vi "Get sub-Array by names.vi"(8 "error in (no error)":errorcluster, 10 "Name Array":string[](array[string]), 11 "JSON Value In":refnum<class "JSON Value.lvclass">) -> (0 "error out":errorcluster, 1 "found":bool, 2 "Array":refnum<class "JSON Value.lvclass">[](array[class]), 3 "JSON Value Out":refnum<class "JSON Value.lvclass">)   [LabVIEW 2020, in "Library Commun.lvlib" / "JSON Value.lvclass"]
doc: "Gets a JSON object from a JSON collection by it's path (an array of strings).\n\nCopyright 2012 James David Powell, Shaun Rumbell and Ton Plomp\nMore information on http://lavag.org/topic/16217-cr-json-labview"
uses:
  JSON Value.lvclass
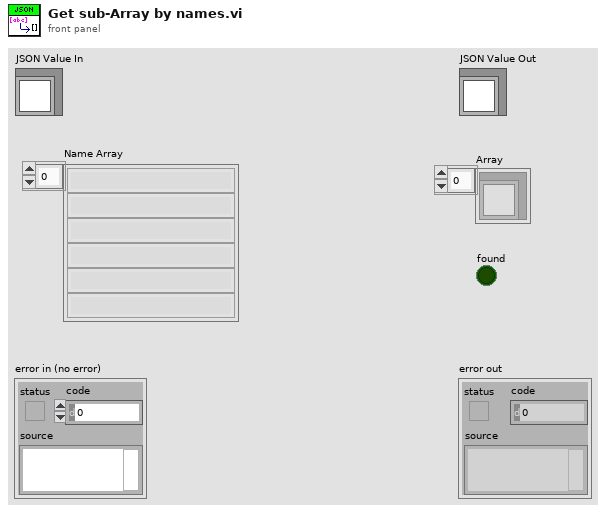
[diagram p1: front panel]
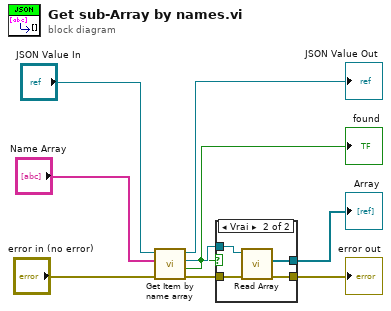
[diagram p0: block diagram]
diagram:
  n1 = call "Get Item by name array.vi"("error in (no error)"="error in (no error)", "Name Array"="Name Array", "JSON Value In"="JSON Value In") -> ("error out"=w2:errorcluster, "found"=w4:bool, "Value"=w5:refnum<class "JSON Value.lvclass">, "JSON Value Out"=→"JSON Value Out":refnum<class "JSON Value.lvclass">)  [unwired: 5 in]
  "found" <- w4
  n2 = case shown="Vrai" w4 {
    tunnel: w5 -> [_ w14]
    tunnel: [_ w13] -> w3
    tunnel: w2 -> [w10 w12]
    tunnel: [w10 w11] -> w1
    frame False {
    }
    frame True {
      n3 = call-dynamic "Read Array.vi"("error in (no error)"=w12, "JSON Value In"=w14) -> ("error out"=w11:errorcluster, "Array"=w13:refnum<class "JSON Value.lvclass">[])  [unwired: 7 in, 1 out]
    }
  }
  "error out" <- w1
  "Array" <- w3
